vi "Pre Launch GUI set-up.vi"(8 "error in (no error)":errorcluster, 10 "GUI ref":refnum<vi>, 11 "Common GUI v3 in":refnum<class "Common GUI v3.lvclass">) -> (0 "error out":errorcluster, 1 "ABORT?":bool, 2 "Circus Logo":picture, 3 "Common GUI v3 out":refnum<class "Common GUI v3.lvclass">)   [LabVIEW 2026, in "TALOS.lvlib" / "Common GUI v3.lvlib" / "Common GUI v3.lvclass"]
uses:
  Common GUI v3.lvclass
  TALOS.lvlib
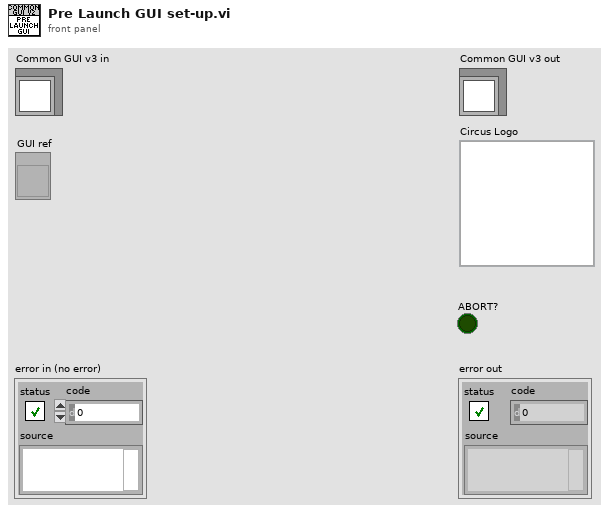
[diagram p1: front panel]
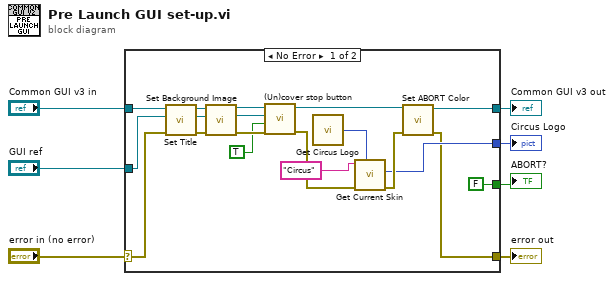
[diagram p0: block diagram]
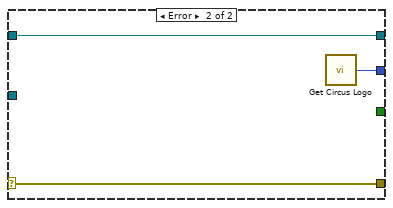
[diagram p2: hidden frame]
diagram:
  n1 = case shown="No Error" "error in (no error)" {
    selector: "error in (no error)" -> [w13 w29]
    tunnel: [w8 w29] -> w6
    tunnel: [w9 w28] -> w4
    tunnel: "Common GUI v3 in" -> [w14 w28]
    tunnel: "GUI ref" -> [w12 _]
    tunnel: [FALSE ("ABORT?") _] -> w2
    tunnel: [w11 w27] -> w1
    frame No Error {
      n2 = call "Set Title.vi"("error in (no error)"=w13, "GUI ref in"=w12, "Common GUI v3 in"=w14) -> ("error out"=w24:errorcluster, "GUI ref out"=w22:refnum<vi>, "Common GUI v3 out"=w23:refnum<class "Common GUI v3.lvclass">)  [unwired: 6 in]
      n3 = call "Set Background Image.vi"("error in (no error)"=w24, "GUI ref in"=w22, "Common GUI v3 in"=w23) -> ("error out"=w20:errorcluster, "GUI ref out"=w19:refnum<vi>, "Common GUI v3 out"=w21:refnum<class "Common GUI v3.lvclass">)  [unwired: 6 in]
      n4 = call-dynamic "(Un)cover stop button.vi"("error in (no error)"=w20, "Cover/Uncover"=TRUE, "GUI ref in"=w19, "Common GUI v3 in"=w21) -> ("error out"=w25:errorcluster, "Common GUI v3 out"=w18:refnum<class "Common GUI v3.lvclass">)  [unwired: 5 in, 1 out]
      n5 = call "Get Circus Logo.vi"() -> ("Circus Logo"=w15:picture)
      n6 = call "Get Current Skin.vi"("default"=w15, "error in (no error)"=w25, "Object"="Circus") -> ("error out"=w26:errorcluster, "Picture with skin"=w11:picture)  [unwired: 3 in, 1 out]
      n7 = call "Set ABORT Color.vi"("error in (no error)"=w26, "Common GUI v3 in"=w18) -> ("error out"=w8:errorcluster, "Common GUI v3 out"=w9:refnum<class "Common GUI v3.lvclass">)  [unwired: 8 in]
    }
    frame Error {
      n8 = call "Get Circus Logo.vi"() -> ("Circus Logo"=w27:picture)
    }
  }
  "error out" <- w6
  "Common GUI v3 out" <- w4
  "ABORT?" <- w2
  "Circus Logo" <- w1
